vi "Write Auto.vi"(8 "error in (no error)":errorcluster, 10 "Auto":T1, 11 "Temperature Controller in":refnum<class "Temperature Controller.lvclass">) -> (0 "error out":errorcluster, 3 "Temperature Controller out":refnum<class "Temperature Controller.lvclass">)   [LabVIEW 2017, in "Temperature Controller.lvclass"]
uses:
  Temperature Controller.lvclass
  AutoCtl.ctl
  Temperature Controller.lvclass/Temperature Controller.ctl
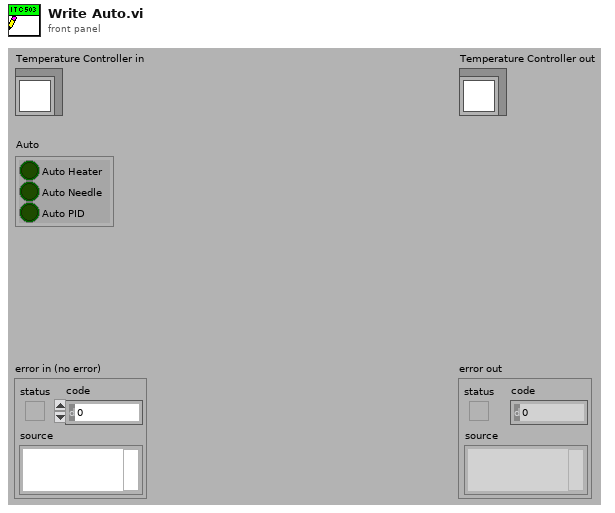
[diagram p1: front panel]
types:
  T1 = typedef "Temperature Controller.lvclass/AutoCtl.ctl" = cluster{"Auto Heater":bool, "Auto Needle":bool, "Auto PID":bool}
  T2 = typedef "ITCIO.ctl" = cluster{"Address":T3, "Version":T4, "Ch 1 dec places":i16, "Ch 2 dec places":i16, "Ch 3 dec places":i16, "Ch1 Name":string, "Ch2 Name":string, "Ch3 Name":string}
  T3 = typedef "OxfordAddress.ctl" = cluster{"Com Port":i32, "ISOBUS Address":i32, "GPIB Address":i16, "Communication":enum16{"RS232", "ISOBUS", "GPIB", "Gateway"}}
  T4 = typedef "ITCVersion.ctl" = enum16{"ITC502", "ITC503", "ITC601"}
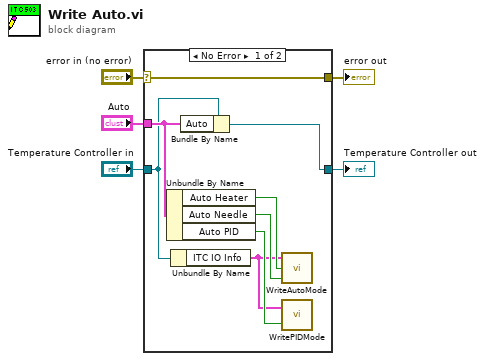
[diagram p0: block diagram]
diagram:
  n1 = case shown="No Error" "error in (no error)" {
    selector: "error in (no error)" -> [w13 w14]
    tunnel: [w13 w14] -> w4
    tunnel: [w12 w15] -> w2
    tunnel: "Temperature Controller in" -> [w7 w15]
    tunnel: "Auto" -> [w8 _]
    frame No Error {
      n2 = Unbundle By Name(w8) -> ("Auto Heater"=w10:bool, "Auto Needle"=w11:bool, "Auto PID"=w9:bool)
      n3 = Unbundle By Name(w7) -> ("ITC IO Info"=w6:T2)
      n4 = Bundle By Name(cluster=w7, "Auto"=w8) -> (w12:refnum<class "Temperature Controller.lvclass">)
      n5 = call "WriteAutoMode.vi"("Auto Needle Valve"=w11, "Auto Heat"=w10, "ITC IO Info"=w6) -> ()  [unwired: 1 out]
      n6 = call "WritePIDMode.vi"("Auto PID"=w9, "ITC IO Info"=w6) -> ()  [unwired: 2 out]
    }
    frame Error {
    }
  }
  "error out" <- w4
  "Temperature Controller out" <- w2
